vi "Add Tree Nodes.vi"(7 "Root path":string, 8 "Event Types":T1[](array[typedef]), 9 "map ref in":map{string, refnum<vi>}(c390), 10 "DQMH Lib In":refnum<vi>, 11 "Tree Map in":T2) -> (1 "map ref out":map{string, refnum<vi>}(c390), 3 "Tree Map out":T2)   [LabVIEW 2020, in "DQMH_API.lvlib"]
uses:
  DQMH_API.lvlib
  <vilib>/National Instruments/Tree Map/Tree Map Data.ctl
  Event types--enum.ctl
  <vilib>/National Instruments/Tree Map/Tree Map.lvlib
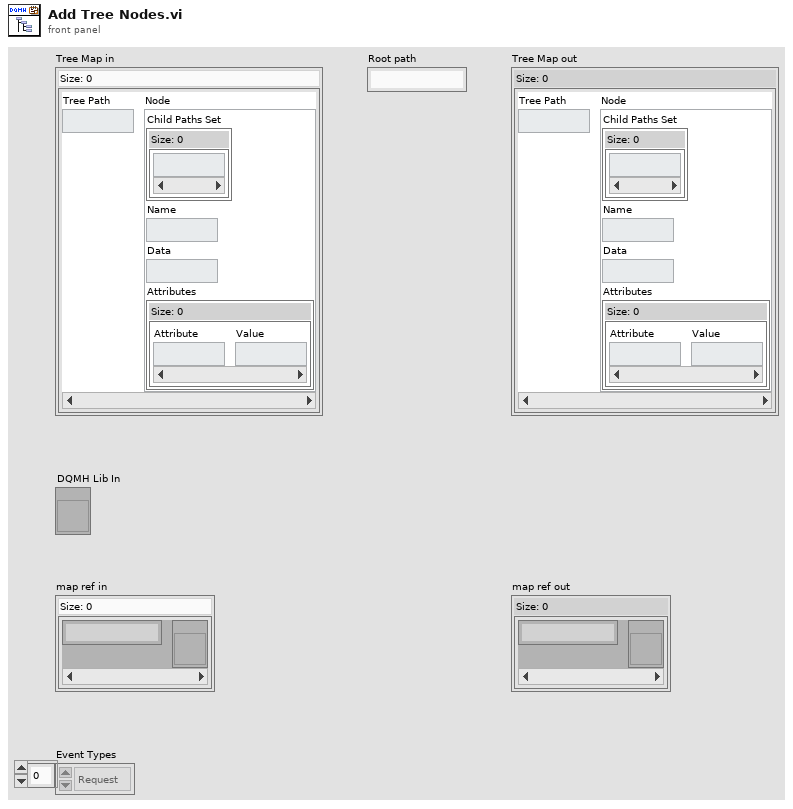
[diagram p1: front panel]
types:
  T1 = typedef "DQMH_API.lvlib/Event types--enum.ctl" = enum16{"Request", "Request and Wait for Reply", "Broadcast"}
  T2 = typedef "Tree Map.lvlib/Tree Map Data.ctl" = map{string, cluster{"Child Paths Set":set{string}, "Name":string, "Data":string, "Attributes":map{string, string}}}
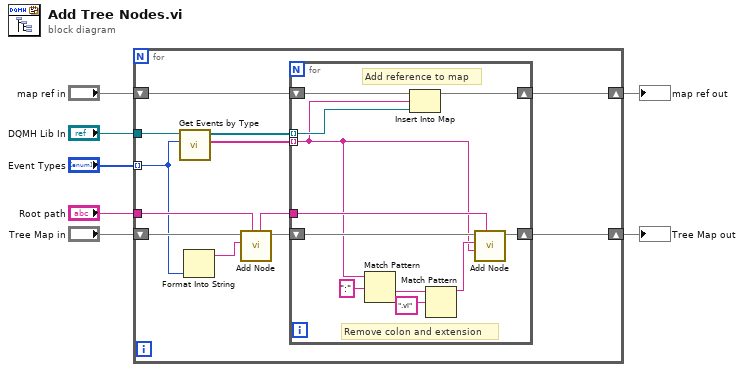
[diagram p0: block diagram]
diagram:
  n1 = for {
    tunnel: "DQMH Lib In" -> [w16]
    tunnel: "Root path" -> [w15]
    tunnel: "Event Types" -> [w8] mode=indexing
    shift-right: [w18] -> w7
    shift-left: "map ref in" -> [w17]
    shift-right: [w14] -> w3
    shift-left: "Tree Map in" -> [w10]
    n2 = call "Get Events by Type.vi"("Event type"=w8, "DQMH Module Ref"=w16) -> ("Event Name"=w13:string[], "Event Ref"=w19:refnum<vi>[])  [unwired: 7 in, 1 out]
    n3 = Format Into String(w8) -> (resulting string=w9:string)  [unwired: 3 in, 1 out]
    n4 = call <vilib>:"Add Node.vi"("Parent Path"=w15, "New Node Name"=w9, "Tree Map In"=w10) -> ("Tree Map Out"=w12:T2, "New Node Path"=w11:string)  [unwired: 6 in, 1 out]
    n5 = for {
      tunnel: w11 -> [w30]
      shift-right: [w28] -> w14
      shift-left: w12 -> [w29]
      tunnel: w13 -> [w20] mode=indexing
      shift-right: [w26] -> w18
      shift-left: w17 -> [w27]
      tunnel: w19 -> [w21] mode=indexing
      # "Add reference to map"
      # "Remove colon and extension"
      n6 = Match Pattern(string=w20, regular expression=":") -> (after substring=w23:string)  [unwired: 1 in, 3 out]
      n7 = Insert Into Map(map in=w27, key=w20, value=w21) -> (map out=w26:map{string, refnum<vi>})  [unwired: 2 out]
      n8 = Match Pattern(string=w23, regular expression=".vi") -> (before substring=w22:string)  [unwired: 1 in, 3 out]
      n9 = call <vilib>:"Add Node.vi"("Parent Path"=w30, "Data"=w20, "New Node Name"=w22, "Tree Map In"=w29) -> ("Tree Map Out"=w28:T2)  [unwired: 5 in, 2 out]
    }
  }
  "map ref out" <- w7
  "Tree Map out" <- w3
